vi "5_Meas_Tr.vi"(0 "file path (IN)":path, 1 "TEST #":string, 5 "ICE":dbl, 7 "Project #":string, 9 "Request #":string, 11 "error in (no error)":errorcluster) -> (2 "Tr (ns)":dbl, 3 "Di/Dt (A/us)":dbl, 4 "file path (OUT)":path, 6 "ON Region":waveform(dbl)[](graph) caption="Tr (ns) & DiDt on (A/us)", 8 "DONE Tr":bool, 10 "DONE Di/Dt ON":bool, 12 "Di (A)":dbl, 13 "Dt (ns)":dbl, 15 "error out":errorcluster)   [LabVIEW 2020]
uses:
  <vilib>/Waveform/WDTOps.llb/WDT Waveform Duration DBL.vi
  <vilib>/Waveform/WDTOps.llb/WDT Get Waveform Subset DBL.vi
  <vilib>/measure/mascope.llb/Transition Measurements 1 chan.vi
  <vilib>/measure/NI_MAPro.lvlib
panel:
  in  "Decision ?":bool
  in  "Cursor b : Channel 1 \nrise edge tolerance":dbl=0.1
  in  "Cursor b : Channel 1 \nrise edge number":i32=1 min=1
  in  "Cursor a : Channel 1 \nrise edge tolerance":dbl=0.1
  in  "Cursor a : Channel 1 \nrise edge number":i32=1 min=1
  out "Cursor b : Channel 1":dbl
  out "Cursor a : Channel 1":dbl
  out "Dt (us)":dbl
  out "90% Ice":dbl
  out "10% Ice":dbl
  out "measurement info (CH1 Cursor a)":T1 {"ref levels"."ref units" items=["absolute", "relative"]; "ref levels"."high ref level" format="%.2p"; "ref levels"."low ref level" format="%.2p"; "ref levels"."mid ref level" format="%.2p"; "end time" format="%.6e"; "start time" format="%.6e"}
  out "measurement info (CH1 Cursor b)":T1 {"ref levels"."ref units" items=["absolute", "relative"]; "ref levels"."high ref level" format="%.2p"; "ref levels"."low ref level" format="%.2p"; "ref levels"."mid ref level" format="%.2p"; "end time" format="%.6e"; "start time" format="%.6e"}
  in  "reference  levels (CH1 2nd Cursor)":T2={"high ref level"=90.0, "mid ref level"=50.0, "low ref level"=10.0, "ref units"=1} {"ref units" items=["absolute", "percent"]; "high ref level" format="%0.2f"; "low ref level" format="%0.2f"; "mid ref level" format="%0.2f"}
  in  "reference  levels (CH1 1st Cursor)":T2={"high ref level"=90.0, "mid ref level"=50.0, "low ref level"=10.0, "ref units"=1} {"ref units" items=["absolute", "percent"]; "high ref level" format="%0.2f"; "low ref level" format="%0.2f"; "mid ref level" format="%0.2f"}
  out "Waveform Graph":waveform(dbl)[](graph)
  # "From 10% Ice to 90% Ice"
  # "Default = 1"
  # "Default = 1"
  # "Default = 0.1"
  # "Default = 0.1"
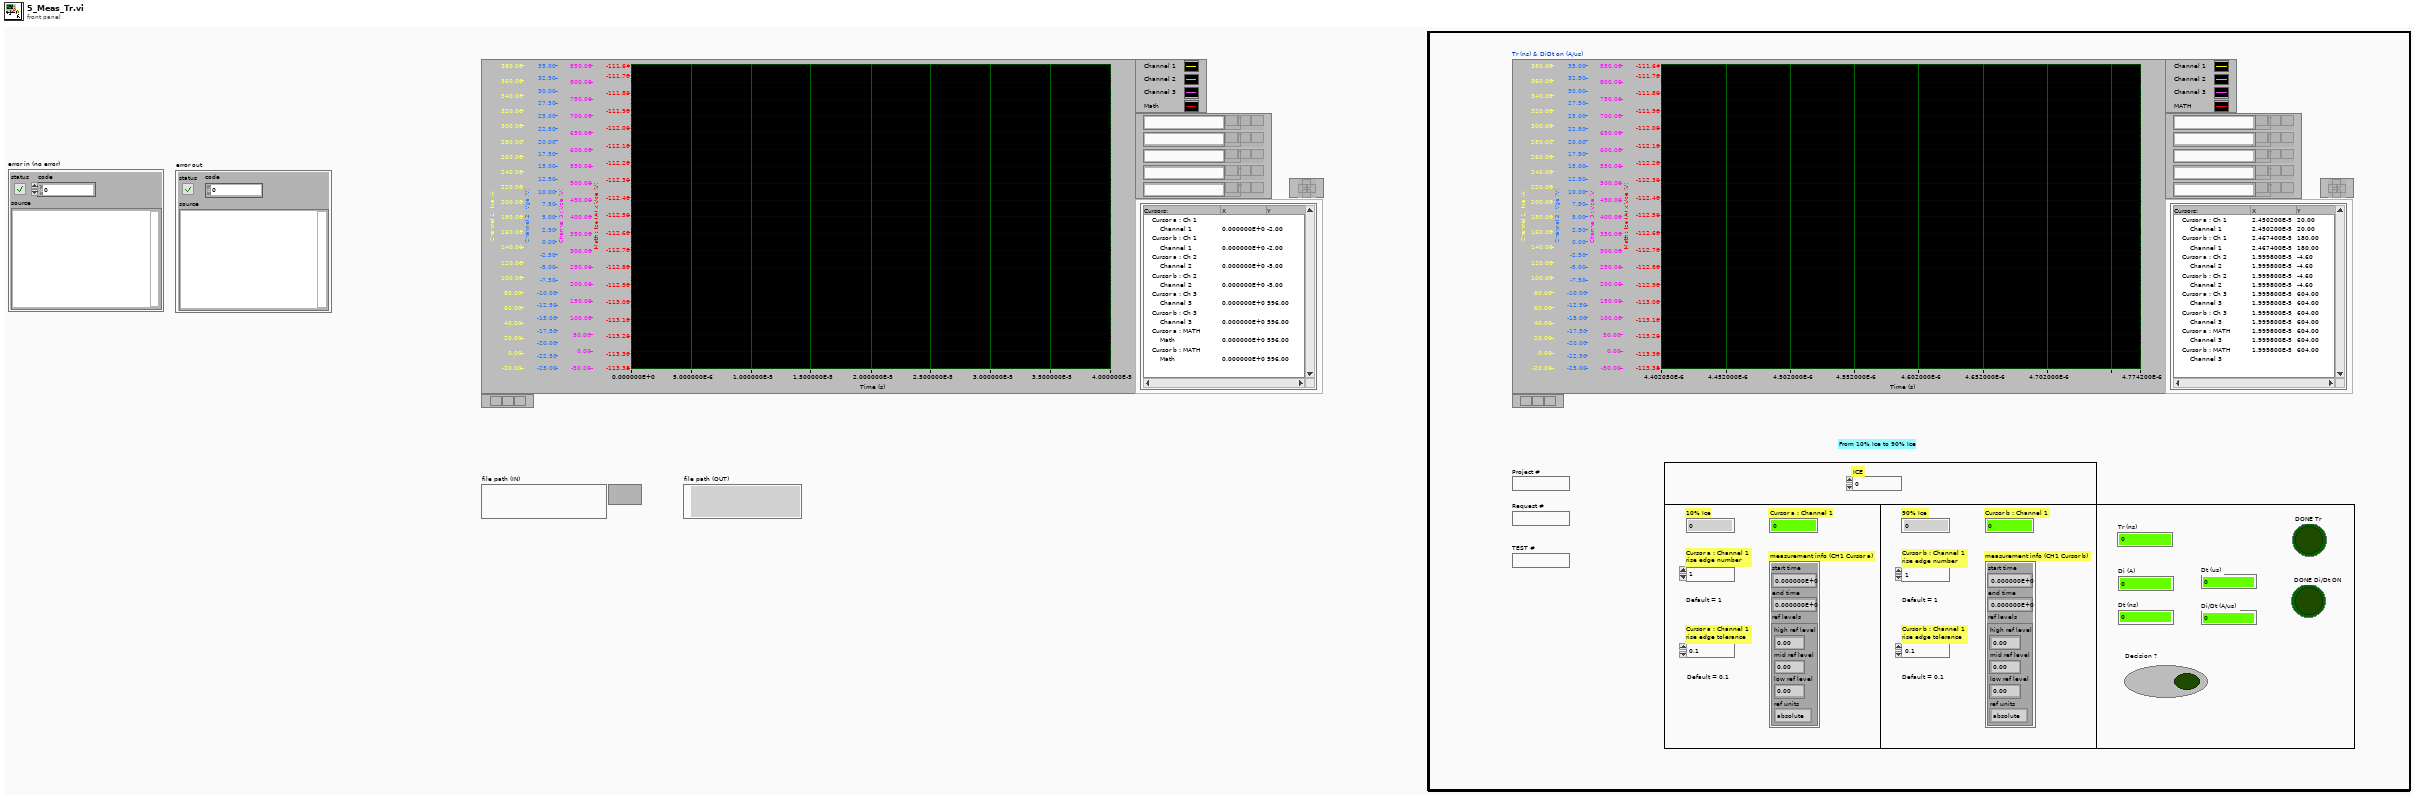
[diagram p1: front panel]
types:
  T1 = cluster{"start time":dbl, "end time":dbl, "ref levels":cluster{"high ref level":dbl, "mid ref level":dbl, "low ref level":dbl, "ref units":u16}}
  T2 = cluster{"high ref level":dbl, "mid ref level":dbl, "low ref level":dbl, "ref units":u16}
  T3 = enum32{"Invalid", "Standard", "Closed", "Hidden", "Minimized", "Maximized"}
  T4 = typedef "imagedata.ctl" = cluster{"image type":i32, "image depth":i32, "image":u8[], "mask":u8[], "colors":u32[], "Rectangle":cluster{"left":i16, "top":i16, "right":i16, "bottom":i16}}
diagram:
  w11 = FALSE ("DONE Tdon")
  w12 = 0.0 ("Cursor a : Channel 1")
  w13 = errorcluster {"status"=FALSE, "code"=0, "source"=""} ("error out")
  w14 = waveform(dbl)[] [] ("Waveform Graph")
  n1 = disable-structure shown="Disabled" {
    frame Disabled {
      n2 = control-ref of="This VI"() -> (w15:refnum<vi>)
      n3 = control-ref of="This VI"() -> (w16:refnum<vi>)
      n4 = invoke class="VI" method="FP.Close"(reference=w15) -> ()  [unwired: 2 in, 3 out]
      n5 = invoke class="VI" method="FP.Open"(reference=w16, "Activate"=TRUE ("Activate?"), "State"=T3."Maximized") -> (error in=w19:errorcluster, error out=w17:errorcluster)  [unwired: 1 in, 4 out]
      n6 = property class="VI"(reference=w16, error in=w17, "Front Panel.Closeable"=TRUE ("Front Panel Window:Closeable")) -> ()  [unwired: 2 out]
    }
    frame Enabled {
    }
  }
  n7 = local write "Cursor a : Channel 1 \nrise edge tolerance"(0.1 ("Cursor a : Channel 1 \nrise edge tolerance")) -> ()
  n8 = local write "Cursor a : Channel 1 \nrise edge number"(1 ("Cursor a : Channel 1 \nrise edge number")) -> ()
  n9 = local write "Cursor b : Channel 1 \nrise edge tolerance"(0.1 ("Cursor b : Channel 1 \nrise edge tolerance")) -> ()
  n10 = local write "Cursor b : Channel 1 \nrise edge number"(1 ("Cursor b : Channel 1 \nrise edge number")) -> ()
  n11 = local write "Cursor a : Channel 1"(w12) -> ()
  n12 = local write "Cursor b : Channel 1"(w12) -> ()
  n13 = local write "DONE Di/Dt ON"(w11) -> ()
  n14 = local write "Decision ?"(w11) -> ()
  n15 = local write "DONE Tr"(w11) -> ()
  n16 = local write "error out"(w13) -> ()
  n17 = local write "error in (no error)"(w13) -> ()
  n18 = local write "Waveform Graph"(w14) -> ()
  n19 = local write "ON Region"(w14) -> ()
  n20 = flat-sequence {
    tunnel: ["file path (IN)"] -> w6
    tunnel: [w22] -> w5
    tunnel: [w31] -> w9
    tunnel: [w30] -> w8
    tunnel: w6 -> [w33]
    tunnel: w5 -> [w32]
    tunnel: [w264] -> w10
    tunnel: w9 -> [w263]
    tunnel: w8 -> [w262]
    tunnel: [w262] -> w7
    tunnel: w10 -> [w279]
    tunnel: w7 -> [w278]
    frame #0 {
      n21 = control-ref of="This VI"() -> (w27:refnum<vi>)
      n22 = invoke class="VI" method="FP.Open"(reference=w27, error in="error in (no error)", "Activate"=TRUE ("Activate?"), "State"=T3."Maximized") -> (error out=w28:errorcluster)  [unwired: 1 in, 4 out]
      n23 = property class="VI"(reference=w27, error in=w28, "Front Panel.Closeable"=TRUE ("Front Panel Window:Closeable")) -> (error out=w22:errorcluster)  [unwired: 1 out]
    }
    frame #1 {
      n24 = while {
        tunnel: w33 -> [w40]
        shift-right: [w35] -> w31
        shift-left: w32 -> [w39]
        tunnel: [w37] -> w30
        stop <- w34 stop-if-true
        n25 = flat-sequence {
          tunnel: [w70] -> w59
          tunnel: [w71] -> w58
          tunnel: w40 -> [w71]
          tunnel: w39 -> [w70]
          tunnel: w59 -> [w163]
          tunnel: w58 -> [w157]
          tunnel: [w86] -> w57
          tunnel: [w85] -> w56
          tunnel: [w75] -> w55
          tunnel: w57 -> [w192]
          tunnel: w56 -> [w206]
          tunnel: [w186] -> w54
          tunnel: w55 -> [w199]
          tunnel: [w199] -> w53
          tunnel: [w176] -> w52
          tunnel: [w185] -> w51
          tunnel: [w184] -> w50
          tunnel: [w183] -> w49
          tunnel: w54 -> [w236]
          tunnel: [w235] -> w48
          tunnel: w53 -> [w237]
          tunnel: [w237] -> w47
          tunnel: w52 -> [w230]
          tunnel: [w230] -> w46
          tunnel: w51 -> [w229]
          tunnel: [w229] -> w45
          tunnel: w50 -> [w227]
          tunnel: [w227] -> w44
          tunnel: w49 -> [w228]
          tunnel: [w228] -> w43
          tunnel: w48 -> [w238]
          tunnel: w47 -> [w251]
          tunnel: [w251] -> w42
          tunnel: w46 -> [w245]
          tunnel: w45 -> [w246]
          tunnel: w44 -> [w244]
          tunnel: w43 -> [w243]
          tunnel: [w238] -> w41
          tunnel: w42 -> [w256]
          tunnel: w41 -> [w258]
          tunnel: [w257] -> w36
          tunnel: [w256] -> w37
          frame #0 {
            w66 = waveform(dbl)[] [] ("Waveform Graph")
            w69 = 0.0 ("Cursor a : Channel 1")
            w68 = FALSE ("DONE Tdon")
            n26 = local write "Cursor a : Channel 1"(w69) -> ()
            n27 = local write "Cursor b : Channel 1"(w69) -> ()
            n28 = local write "DONE Di/Dt ON"(w68) -> ()
            n29 = local write "Decision ?"(w68) -> ()
            n30 = local write "DONE Tr"(w68) -> ()
            n31 = Wait (ms)(milliseconds to wait=u32 200) -> ()  [unwired: 1 out]
            n32 = local write "Waveform Graph"(w66) -> ()
            n33 = local write "ON Region"(w66) -> ()
          }
          frame #1 {
            w138 = u16 1 items=["Samples", "Relative Time"] ("start/duration format")
            w149 = u16 1 items=["Samples", "Relative Time"] ("start/duration format")
            w150 = u16 1 items=["Samples", "Relative Time"] ("start/duration format")
            # "Channel 1"
            # "Channel 3"
            # "Channel 2"
            # "dt"
            # "Ch2"
            # "Ch1"
            n34 = call "3_ReadDatatoWaveform.vi"("error in (no error)"=w163, "file path (IN)"=w157) -> ("error out"=w131:errorcluster, "Waveform Graph"=→"Waveform Graph":waveform(dbl)[], "file path (OUT)"=w75:path, "dt"=w158:dbl, "Ch 2 Data"=w155:dbl[], "Ch 3 Data"=w159:dbl[], "Ch 1 Data"=w156:dbl[])  [unwired: 3 in]
            n35 = To Time Stamp(1:0.0 ("number")) -> (0:w160:timestamp)
            n36 = disable-structure shown="Enabled" {
              disable-tunnel: w160 -> [w167 _]
              disable-tunnel: w158 -> [w166 _]
              disable-tunnel: w156 -> [w165 _]
              disable-tunnel: [w164 _] -> w137
              frame Enabled {
                # "Channel 1"
                n37 = Bundle By Name("Y"=w165, "dt"=w166, "t0"=w167) -> (w164:waveform(dbl))  [unwired: 1 in]
              }
              frame Disabled {
              }
            }
            n38 = disable-structure shown="Enabled" {
              disable-tunnel: w160 -> [w171 _]
              disable-tunnel: w158 -> [w170 _]
              disable-tunnel: w155 -> [w169 _]
              disable-tunnel: [w168 _] -> w136
              frame Enabled {
                # "Channel 2"
                n39 = Bundle By Name("Y"=w169, "dt"=w170, "t0"=w171) -> (w168:waveform(dbl))  [unwired: 1 in]
              }
              frame Disabled {
              }
            }
            n40 = disable-structure shown="Enabled" {
              disable-tunnel: w160 -> [w175 _]
              disable-tunnel: w158 -> [w174 _]
              disable-tunnel: w159 -> [w173 _]
              disable-tunnel: [w172 _] -> w135
              frame Enabled {
                # "Channel 3"
                n41 = Bundle By Name("Y"=w173, "dt"=w174, "t0"=w175) -> (w172:waveform(dbl))  [unwired: 1 in]
              }
              frame Disabled {
              }
            }
            n42 = call-poly <vilib>:"Waveform Duration.vi"("error in (no error)"=w131, "waveform in"=w135) -> ("error out"=w143:errorcluster, "duration"=w140:dbl, "waveform out"=w142:waveform(dbl))  [unwired: 7 in]
            n43 = call-poly <vilib>:"Waveform Duration.vi"("error in (no error)"=w131, "waveform in"=w136) -> ("error out"=w144:errorcluster, "duration"=w147:dbl, "waveform out"=w145:waveform(dbl))  [unwired: 7 in]
            n44 = call-poly <vilib>:"Waveform Duration.vi"("error in (no error)"=w131, "waveform in"=w137) -> ("error out"=w154:errorcluster, "duration"=w151:dbl, "waveform out"=w153:waveform(dbl))  [unwired: 7 in]
            n45 = Divide(x=w140, y=2.0) -> (x/y=w139:dbl)
            n46 = Divide(x=w147, y=2.0) -> (x/y=w148:dbl)
            n47 = Divide(x=w151, y=2.0) -> (x/y=w132:dbl)
            n48 = call-poly <vilib>:"Get Waveform Subset.vi"("start/duration format"=w138, "error in (no error)"=w143, "duration"=w139, "start samples/time"=w139, "waveform in"=w142) -> ("error out"=w128:errorcluster, "waveform out"=w134:waveform(dbl))  [unwired: 1 in, 2 out]
            n49 = call-poly <vilib>:"Get Waveform Subset.vi"("start/duration format"=w149, "error in (no error)"=w144, "duration"=w148, "start samples/time"=w148, "waveform in"=w145) -> ("error out"=w129:errorcluster, "waveform out"=w87:waveform(dbl))  [unwired: 1 in, 2 out]
            n50 = call-poly <vilib>:"Get Waveform Subset.vi"("start/duration format"=w150, "error in (no error)"=w154, "duration"=w132, "start samples/time"=w132, "waveform in"=w153) -> ("error out"=w130:errorcluster, "waveform out"=w86:waveform(dbl))  [unwired: 1 in, 2 out]
            n51 = Build Array(w86, w87, w134) -> (→"ON Region":waveform(dbl)[])
            n52 = Merge Errors(w130, w129, w128) -> (w83:errorcluster)
            n53 = property on="ON Region" class="WFGraph (strict)"(error in=w83) -> (error out=w82:errorcluster, "Width"=w81:u32)  [unwired: 1 in, 1 out]
            n54 = property on="ON Region" class="WFGraph (strict)"(error in=w82, "Caption.Justify"=enum16{"Left", "Center", "Right"}."Left" ("Caption.Justification"), "Caption.Width"=w81, "Caption.FontBold"=TRUE ("Caption.Font:Bold"), "Caption.FontColor"=u32 16860 ("Caption.Font:Color"), "Caption.FontSize"=u32 24 ("Caption.Font:Size"), "Caption.Text"="Tr (ns) & DiDt on (A/us)") -> (error out=w77:errorcluster)  [unwired: 1 in, 1 out]
            n55 = property on="ON Region" class="WFGraph (strict)"(error in=w77, "XScale.Offset"=w132) -> (error out=w111:errorcluster)  [unwired: 1 in, 1 out]
            n56 = property on="ON Region" class="WFGraph (strict)"(error in=w111, "Active Cursor"=u32 0, "Cursor.Cursor X"=0.0 ("Cursor.Cursor Position:Cursor X"), "Cursor.Cursor Y"=0.0 ("Cursor.Cursor Position:Cursor Y"), "Cursor.Visible"=FALSE) -> (error out=w110:errorcluster)  [unwired: 1 in, 1 out]
            n57 = property on="ON Region" class="WFGraph (strict)"(error in=w110, "Active Cursor"=u32 1, "Cursor.Cursor X"=0.0 ("Cursor.Cursor Position:Cursor X"), "Cursor.Cursor Y"=0.0 ("Cursor.Cursor Position:Cursor Y"), "Cursor.Visible"=FALSE) -> (error out=w109:errorcluster)  [unwired: 1 in, 1 out]
            n58 = property on="ON Region" class="WFGraph (strict)"(error in=w109, "Active Cursor"=u32 2, "Cursor.Cursor X"=0.0 ("Cursor.Cursor Position:Cursor X"), "Cursor.Cursor Y"=0.0 ("Cursor.Cursor Position:Cursor Y"), "Cursor.Visible"=FALSE) -> (error out=w108:errorcluster)  [unwired: 1 in, 1 out]
            n59 = property on="ON Region" class="WFGraph (strict)"(error in=w108, "Active Cursor"=u32 3, "Cursor.Cursor X"=0.0 ("Cursor.Cursor Position:Cursor X"), "Cursor.Cursor Y"=0.0 ("Cursor.Cursor Position:Cursor Y"), "Cursor.Visible"=FALSE) -> (error out=w91:errorcluster)  [unwired: 1 in, 1 out]
            n60 = property on="ON Region" class="WFGraph (strict)"(error in=w91, "Active Cursor"=u32 4, "Cursor.Cursor X"=0.0 ("Cursor.Cursor Position:Cursor X"), "Cursor.Cursor Y"=0.0 ("Cursor.Cursor Position:Cursor Y"), "Cursor.Visible"=FALSE) -> (error out=w90:errorcluster)  [unwired: 1 in, 1 out]
            n61 = property on="ON Region" class="WFGraph (strict)"(error in=w90, "Active Cursor"=u32 5, "Cursor.Cursor X"=0.0 ("Cursor.Cursor Position:Cursor X"), "Cursor.Cursor Y"=0.0 ("Cursor.Cursor Position:Cursor Y"), "Cursor.Visible"=FALSE) -> (error out=w89:errorcluster)  [unwired: 1 in, 1 out]
            n62 = property on="ON Region" class="WFGraph (strict)"(error in=w89, "Active Cursor"=u32 6, "Cursor.Cursor X"=0.0 ("Cursor.Cursor Position:Cursor X"), "Cursor.Cursor Y"=0.0 ("Cursor.Cursor Position:Cursor Y"), "Cursor.Visible"=FALSE) -> (error out=w88:errorcluster)  [unwired: 1 in, 1 out]
            n63 = property on="ON Region" class="WFGraph (strict)"(error in=w88, "Active Cursor"=u32 7, "Cursor.Cursor X"=0.0 ("Cursor.Cursor Position:Cursor X"), "Cursor.Cursor Y"=0.0 ("Cursor.Cursor Position:Cursor Y"), "Cursor.Visible"=FALSE) -> (error out=w85:errorcluster)  [unwired: 1 in, 1 out]
            n64 = call <vilib>:"Beep.vi"("use system alert? (T)"=FALSE, "duration (msec)"=u32 200, "frequency (Hz)"=u32 2000) -> ()  [unwired: 9 in]
          }
          frame #2 {
            w219 = u16 1 items=["falling", "rising"] ("polarity (rising)")
            w220 = u16 1 items=["falling", "rising"] ("polarity (rising)")
            # "Cursor a : Channel 1"
            # "Cursor b : Channel 1"
            # "Cursor b : Channel 1"
            # "Cursor a : Channel 1"
            # "Cursor b : Channel 1"
            # "Cursor a : Channel 1"
            # "Cursor b : Channel 1"
            # "Cursor a : Channel 1"
            # "End Time 1st Cursor"
            # "End Time 2nd Cursor"
            # "1st PARAMETER : 10% Ice"
            # "Channel 1"
            # "2nd PARAMETER : 90% Ice"
            # "Channel 1"
            n65 = Divide(x=10.0, y=100.0) -> (x/y=w226:dbl)
            n66 = Multiply(x=w226, y="ICE") -> (x*y=w194:dbl)
            "10% Ice" <- w194
            n67 = Add(x=w194, y="Cursor a : Channel 1 \nrise edge tolerance") -> (x+y=w212:dbl)
            n68 = Subtract(x=w194, y="Cursor a : Channel 1 \nrise edge tolerance") -> (x-y=w211:dbl)
            n69 = Bundle By Name(cluster="reference  levels (CH1 1st Cursor)", "high ref level"=w212, "mid ref level"=w194, "low ref level"=w211, "ref units"=u16 0) -> (w208:T2)
            n70 = call-poly <vilib>:"Transition Measurements.vi"("edge number (1)"="Cursor a : Channel 1 \nrise edge number", "error in (no error)"=w206, "reference levels"=w208, "polarity (rising)"=w220, "signal in"=w192) -> ("error out"=w203:errorcluster, "measurement info"=w207:T1)  [unwired: 1 in, 4 out]
            "measurement info (CH1 Cursor a)" <- w207
            n71 = Unbundle By Name(w207) -> ("end time"=w183:dbl)
            n72 = property on="ON Region" class="WFGraph (strict)"(error in=w203, "Active Cursor"=u32 0, "Cursor.Cursor X"=w183, "Cursor.Visible"=TRUE, "Cursor.Cursor Name Visible"=TRUE) -> (error out=w191:errorcluster)  [unwired: 1 in, 1 out]
            n73 = property on="ON Region" class="WFGraph (strict)"(error in=w191, "Active Cursor"=u32 0) -> (error out=w189:errorcluster, "Cursor.Cursor Y"=w176:dbl)  [unwired: 1 in, 1 out]
            "Cursor a : Channel 1" <- w176
            n74 = Divide(x=90.0, y=100.0) -> (x/y=w223:dbl)
            n75 = Multiply(x=w223, y="ICE") -> (x*y=w195:dbl)
            "90% Ice" <- w195
            n76 = Add(x=w195, y="Cursor b : Channel 1 \nrise edge tolerance") -> (x+y=w218:dbl)
            n77 = Subtract(x=w195, y="Cursor b : Channel 1 \nrise edge tolerance") -> (x-y=w217:dbl)
            n78 = Bundle By Name(cluster="reference  levels (CH1 2nd Cursor)", "high ref level"=w218, "mid ref level"=w195, "low ref level"=w217, "ref units"=u16 0) -> (w214:T2)
            n79 = call-poly <vilib>:"Transition Measurements.vi"("edge number (1)"="Cursor b : Channel 1 \nrise edge number", "error in (no error)"=w189, "reference levels"=w214, "polarity (rising)"=w219, "signal in"=w192) -> ("error out"=w200:errorcluster, "measurement info"=w213:T1)  [unwired: 1 in, 4 out]
            "measurement info (CH1 Cursor b)" <- w213
            n80 = Unbundle By Name(w213) -> ("end time"=w184:dbl)
            n81 = property on="ON Region" class="WFGraph (strict)"(error in=w200, "Active Cursor"=u32 1, "Cursor.Cursor X"=w184, "Cursor.Visible"=TRUE, "Cursor.Cursor Name Visible"=TRUE) -> (error out=w187:errorcluster)  [unwired: 1 in, 1 out]
            n82 = call <vilib>:"Beep.vi"("use system alert? (T)"=FALSE, "duration (msec)"=u32 200, "frequency (Hz)"=u32 2000) -> ()  [unwired: 9 in]
            n83 = property on="ON Region" class="WFGraph (strict)"(error in=w187, "Active Cursor"=u32 1) -> (error out=w186:errorcluster, "Cursor.Cursor Y"=w185:dbl)  [unwired: 1 in, 1 out]
            "Cursor b : Channel 1" <- w185
          }
          frame #3 {
            # "2nd Cursor"
            # "1st Cursor"
            n84 = Subtract(x=w228, y=1e-07) -> (x-y=w231:dbl)
            n85 = Add(x=w227, y=1e-07) -> (x+y=w232:dbl)
            n86 = property on="ON Region" class="WFGraph (strict)"(error in=w236, "XScale.Minimum"=w231, "XScale.Maximum"=w232) -> (error out=w235:errorcluster)  [unwired: 1 in, 1 out]
          }
          frame #4 {
            # "us"
            # "ns"
            n87 = Subtract(x=w246, y=w245) -> (x-y=w241:dbl)
            n88 = Subtract(x=w244, y=w243) -> (x-y=w242:dbl)
            n89 = Absolute Value(x=w241) -> (abs(x)=w240:dbl)
            "Di (A)" <- w240
            n90 = Absolute Value(x=w242) -> (abs(x)=w239:dbl)
            n91 = Multiply(x=w239, y=1000000000.0) -> (x*y=→"Tr (ns)" →"Dt (ns)":dbl)
            n92 = Multiply(x=w239, y=1000000.0) -> (x*y=w248:dbl)
            "Dt (us)" <- w248
            n93 = call <vilib>:"Beep.vi"("use system alert? (T)"=FALSE, "duration (msec)"=u32 200, "frequency (Hz)"=u32 2000) -> ()  [unwired: 9 in]
            n94 = Divide(x=w240, y=w248) -> (x/y=→"Di/Dt (A/us)":dbl)
          }
          frame #5 {
            n95 = while {
              shift-right: [w259] -> w257
              shift-left: w258 -> [w259]
              stop <- "Decision ?" stop-if-true
              n96 = Wait (ms)(milliseconds to wait=u32 100) -> ()  [unwired: 1 out]
            }
          }
        }
        n97 = while {
          tunnel: [w61] -> w34
          shift-right: [w64] -> w35
          shift-left: w36 -> [w65]
          stop <- w63 stop-if-true
          n98 = Wait (ms)(milliseconds to wait=u32 100) -> ()  [unwired: 1 out]
          n99 = call "Display Message to User"("error in (no error)"=w65) -> ("error out"=w64:errorcluster, "NO"=w61:bool)  [unwired: 9 in]
          n100 = Or(x=w61, y=TRUE) -> (x .or. y?=w63:bool)
        }
        n101 = Wait (ms)(milliseconds to wait=u32 100) -> ()  [unwired: 1 out]
      }
    }
    frame #2 {
      w267 = "_"
      n102 = invoke on="ON Region" class="WFGraph (strict)" method="Get Image"(error in=w263) -> (error out=w271:errorcluster, "image data"=w274:T4)  [unwired: 5 in, 4 out]
      n103 = Concatenate Strings("C:\\Inductive_Switching_Project\\IndSw_Image\\" ("string"), "Project #", w267, "Request #", w267, "TEST #", w267, "Tr_DiDton" ("string"), ".png" ("string")) -> (w275:string)
      n104 = String To Path(string=w275) -> (path=w273:path)
      n105 = call <vilib>:"Write PNG File.vi"("error in (no error)"=w271, "image data"=w274, "path to PNG file"=w273) -> ("error out"=w264:errorcluster)  [unwired: 7 in, 1 out]
      "DONE Tr" <- TRUE ("DONE Tdon")
      "DONE Di/Dt ON" <- TRUE ("DONE Di/Dt ON")
    }
    frame #3 {
      n106 = disable-structure shown="Enabled" {
        disable-tunnel: w279 -> [w280 _]
        frame Enabled {
          n107 = control-ref of="This VI"() -> (w281:refnum<vi>)
          n108 = invoke class="VI" method="FP.Close"(reference=w281, error in=w280) -> ()  [unwired: 1 in, 3 out]
        }
        frame Disabled {
        }
      }
      "error out" <- w279
      "file path (OUT)" <- w278
    }
  }
